vi "Application_Init.vi"(0 "object in":refnum<class "Application.lvclass">, 5 "error in (no error)":errorcluster) -> (14 "object out":refnum<class "Application.lvclass">, 19 "error out":errorcluster)   [LabVIEW 2021, in "Application.lvclass"]
uses:
  Application.lvclass
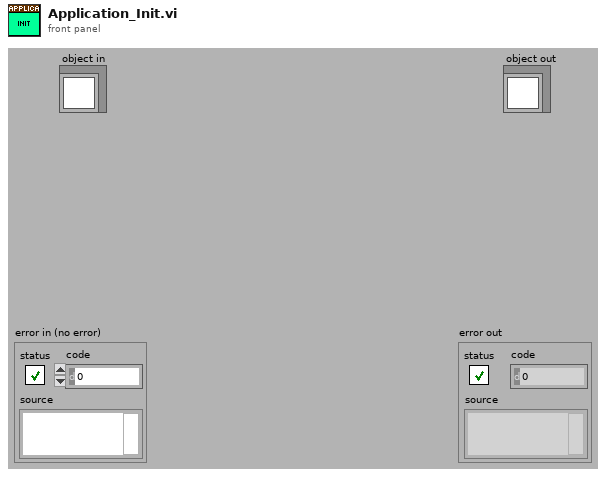
[diagram p1: front panel]
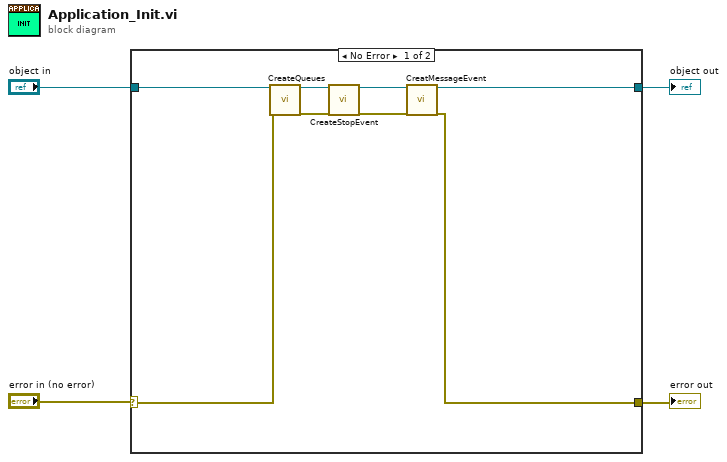
[diagram p0: block diagram]
diagram:
  n1 = case shown="No Error" "error in (no error)" {
    selector: "error in (no error)" -> [w10 w13]
    tunnel: "object in" -> [w9 w14]
    tunnel: [w7 w14] -> w3
    tunnel: [w5 w13] -> w1
    frame No Error {
      n2 = call-dynamic "CreateQueues.vi"("object in"=w9, "error in (no error)"=w10) -> ("object out"=w12:refnum<class "Application.lvclass">, "error out"=w11:errorcluster)  [unwired: 16 in]
      n3 = call "CreateStopEvent.vi"("object in"=w12, "error in (no error)"=w11) -> ("object out"=w8:refnum<class "Application.lvclass">, "error out"=w6:errorcluster)  [unwired: 16 in]
      n4 = call "CreatMessageEvent.vi"("object in"=w8, "error in (no error)"=w6) -> ("object out"=w7:refnum<class "Application.lvclass">, "error out"=w5:errorcluster)  [unwired: 16 in]
    }
    frame Error {
    }
  }
  "object out" <- w3
  "error out" <- w1
